vi "Set Slew Rates.vi"(0 "object in":refnum<class "HPS-17000-PowerModule.lvclass">, 5 "Slew Rates":T1, 11 "Error In":errorcluster) -> (4 "object out":refnum<class "HPS-17000-PowerModule.lvclass">, 15 "Error Out":errorcluster)   [LabVIEW 2023, in "HPS-17000-PowerModule.lvlib" / "HPS-17000-PowerModule.lvclass"]
uses:
  HPS-17000-PowerModule.lvclass
  builds/PowerModuleInterface/PowerModuleInterface.lvlibp/Classes/PowerModule_interface/Slew Rates.ctl
  builds/PowerModuleInterface/PowerModuleInterface.lvlibp/Classes/PowerModule_interface/PowerModuleInterface.lvclass
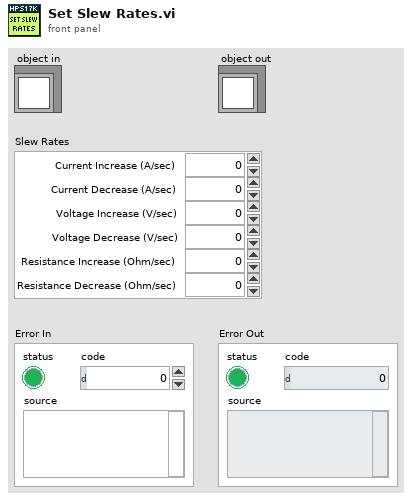
[diagram p1: front panel]
types:
  T1 = typedef "PowerModuleInterface.lvlibp/PowerModuleInterface.lvclass/Slew Rates.ctl" = cluster{"Current Decrease (A/sec)":dbl, "Current Increase (A/sec)":dbl, "Voltage Decrease (V/sec)":dbl, "Voltage Increase (V/sec)":dbl, "Resistance Decrease (Ohm/sec)":dbl, "Resistance Increase (Ohm/sec)":dbl}
  T2 = typedef "HPS-17000-PowerModule.lvlib/HPS-17000-PowerModule.lvclass/ObjectAttributes.ctl" = cluster{"JSON Config Path":path, "Configuration":T3, "GM ID":string, "HPS17000 Refs":refnum<class "HPS-17000.lvclass">[], "connected":bool, "reserved":bool, "events":T5, "nibatterycycler_grpc_Setpoint":T6, "last timestamp":i64, "mode":T7, "range":T8, "measurement array":T9[]}
  T3 = typedef "HPS-17000-PowerModule.lvlib/HPS-17000-PowerModule.lvclass/Configuration.ctl" = cluster{"TSN NIC IP Address":string, "HPS17000 IP Addresses":string[], "HPS Topology":enum16{"SINGLE", "MULTI"}, "Setpoint Stream Config":T4, "Measurement Array Size":i32}
  T4 = typedef "Cycler.lvclass/Setpoint Stream Basic Config.ctl" = cluster{"local address":string, "receiver port":u16}
  T5 = typedef "HPS-17000.lvclass/Multi-Cycler Events.ctl" = cluster{"heartbeats events":refnum<user-event>[], "faults events":refnum<user-event>[], "network sync event":refnum<user-event>[], "setpoint status event":refnum<user-event>[]}
  T6 = typedef "NI_BC_client.lvlib/nibatterycycler_grpc_Setpoint.ctl" = cluster{"voltage":sgl, "current":sgl, "min_power":sgl, "max_power":sgl, "resistance":sgl}
  T7 = typedef "HPS-17000-PowerModule.lvlib/HPS-17000-PowerModule.lvclass/Mode.ctl" = u16
  T8 = typedef "PowerModuleInterface.lvlibp/PowerModuleInterface.lvclass/Range.ctl" = cluster{"Current Max (A)":dbl, "Current Min (A)":dbl, "Voltage Max (V)":dbl, "Voltage Min (V)":dbl}
  T9 = typedef "PowerModuleInterface.lvlibp/PowerModuleInterface.lvclass/Measurements.ctl" = cluster{"measured voltage (V)":dbl, "measured current (A)":dbl, "setpoint voltage (V)":dbl, "setpoint current (A)":dbl, "timestamp":dbl}
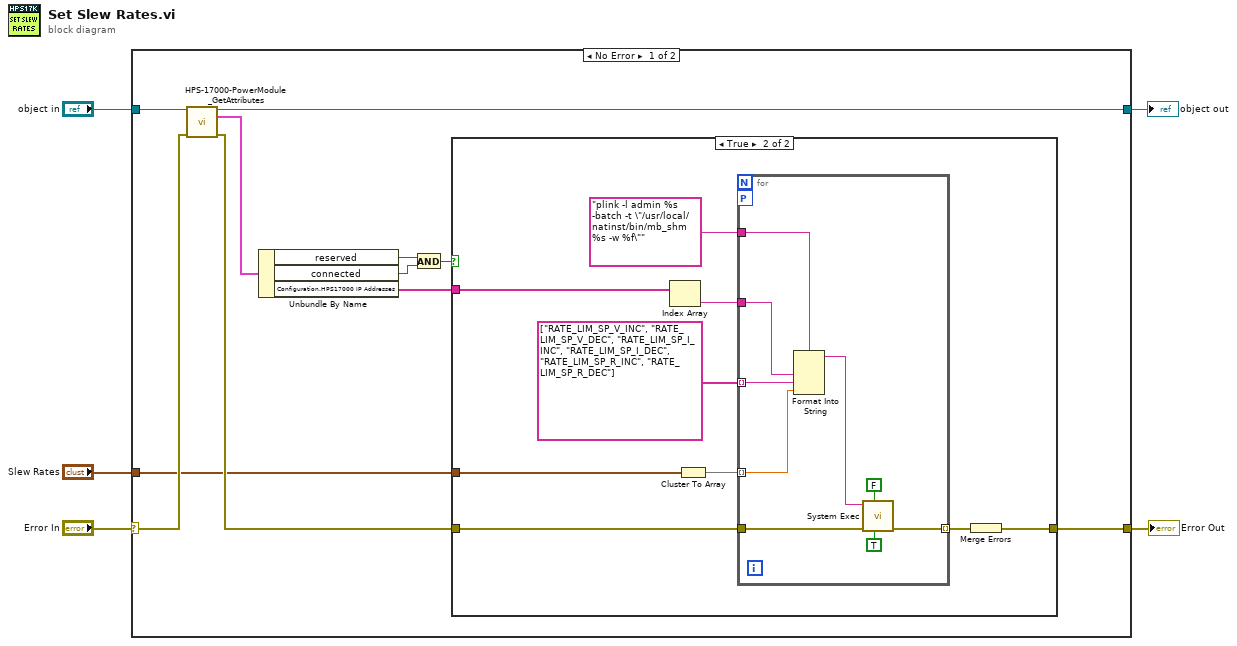
[diagram p0: block diagram]
diagram:
  n1 = case shown="No Error" "Error In" {
    selector: "Error In" -> [w13 w36]
    tunnel: [w16 w36] -> w3
    tunnel: "object in" -> [w15 w37]
    tunnel: [w14 w37] -> w4
    tunnel: "Slew Rates" -> [w6 _]
    frame No Error {
      n2 = call "HPS-17000-PowerModule_GetAttributes.vi"("reference in"=w15, "Error In"=w13) -> ("reference out"=w14:refnum<class "HPS-17000-PowerModule.lvclass">, "Data"=w11:T2, "Error Out"=w12:errorcluster)  [unwired: 10 in, 1 out]
      n3 = Unbundle By Name(w11) -> ("reserved"=w9:bool, "connected"=w8:bool, "Configuration.HPS17000 IP Addresses"=w10:string[])
      n4 = And(x=w9, y=w8) -> (x .and. y?=w7:bool)
      n5 = case shown="True" w7 {
        tunnel: [w17 w24] -> w16
        tunnel: w12 -> [w17 w23]
        tunnel: w10 -> [_ w22]
        tunnel: w6 -> [_ w19]
        frame False {
        }
        frame True {
          n6 = Index Array(array=w22) -> (element=w21:string)  [unwired: 1 in]
          n7 = Cluster To Array(cluster=w19) -> (array=w18:dbl[])
          n8 = for {
            tunnel: w23 -> [w33]
            tunnel: [w29] -> w25 mode=indexing
            tunnel: "plink -l admin %s -batch -t \"/usr/local/natinst/bin/mb_shm %s -w %f\"" ("format string") -> [w32]
            tunnel: string[] ["RATE_LIM_SP_V_INC", "RATE_LIM_SP_V_DEC", "RATE_LIM_SP_I_INC", "RATE_LIM_SP_I_DEC", "RATE_LIM_SP_R_INC", "RATE_LIM_SP_R_DEC"] -> [w30] mode=indexing
            workers-P: _ -> [_]
            tunnel: w21 -> [w28]
            tunnel: w18 -> [w27] mode=indexing
            n9 = Format Into String(format string=w32, w28, w30, w27) -> (resulting string=w31:string)  [unwired: 2 in, 1 out]
            n10 = call <vilib>:"System Exec.vi"("run minimized? (F)"=TRUE, "wait until completion? (T)"=FALSE, "error in (no error)"=w33, "command line"=w31) -> ("error out"=w29:errorcluster)  [unwired: 4 in, 3 out]
          }
          n11 = Merge Errors(w25) -> (w24:errorcluster)
        }
      }
    }
    frame Error {
    }
  }
  "Error Out" <- w3
  "object out" <- w4
